vi "Create Top Level.vi"(9 "Alias":string, 10 "Actor":refnum<class "Actor.lvclass">) -> ()   [LabVIEW 2021, in "LVCAM.lvlib" / "Self Actor.lvclass"]
uses:
  Self Actor.lvclass
  Actor/Actor.lvclass
  Self Actor.lvclass/Self Actor.ctl
  LVCAM.lvlib
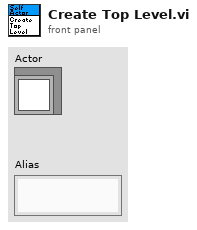
[diagram p1: front panel]
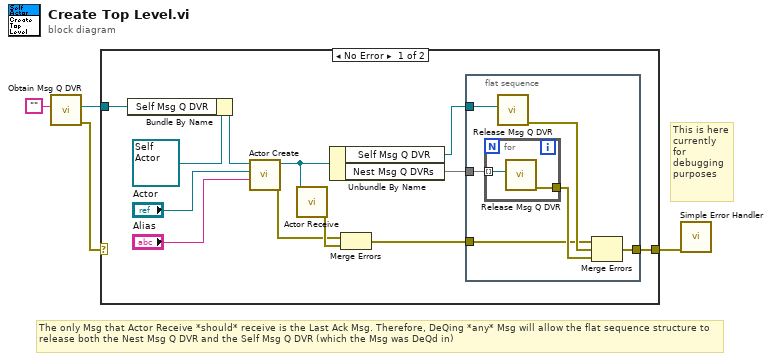
[diagram p0: block diagram]
diagram:
  # "This is here currently for debugging purposes"
  # "The only Msg that Actor Receive *should* receive is the Last Ack Msg. Therefore, DeQing *any* Msg will allow the flat sequence structure to release both the Nest Msg Q DVR and the Self Msg Q DVR (which the Msg was DeQd in)"
  n1 = call "Obtain Msg Q DVR.vi"("Msg Q DVR Alias"="") -> ("error out"=w1:errorcluster, "Msg Q DVR"=w4:refnum<data-value>)  [unwired: 9 in]
  n2 = case shown="No Error" w1 {
    selector: w1 -> [_ w25]
    tunnel: w4 -> [w15 _]
    tunnel: [w14 w25] -> w3
    frame No Error {
      n3 = Bundle By Name(cluster=refnum<class "Self Actor.lvclass"> refnum ("Self Actor in"), "Self Msg Q DVR"=w15) -> (w11:refnum<class "Self Actor.lvclass">)
      n4 = call-dynamic "Actor Create.vi"("Nest Alias"="Alias", "Nest Actor"="Actor", "Self Actor in"=w11) -> ("error out"=w5:errorcluster, "Self Actor out"=w7:refnum<class "Self Actor.lvclass">)  [unwired: 7 in]
      n5 = call-dynamic "Actor Receive.vi"("Self Actor in"=w7) -> ("error out"=w6:errorcluster)  [unwired: 8 in, 2 out]
      n6 = Unbundle By Name(w7) -> ("Self Msg Q DVR"=w16:refnum<data-value>, "Nest Msg Q DVRs"=w13:set{refnum<data-value>})
      n7 = Merge Errors(w5, w6) -> (w12:errorcluster)
      n8 = flat-sequence {
        tunnel: w16 -> [w22]
        tunnel: [w21] -> w14
        tunnel: w13 -> [w20]
        tunnel: w12 -> [w17]
        frame #0 {
          n9 = for {
            tunnel: w20 -> [w24] mode=indexing
            tunnel: [w23] -> w19
            n10 = call "Release Msg Q DVR.vi"("Msg Q DVR"=w24) -> ("error out"=w23:errorcluster)  [unwired: 10 in]
          }
          n11 = call "Release Msg Q DVR.vi"("Msg Q DVR"=w22) -> ("error out"=w18:errorcluster)  [unwired: 10 in]
          n12 = Merge Errors(w17, w18, w19) -> (w21:errorcluster)
        }
      }
    }
    frame Error {
    }
  }
  n13 = call <vilib>:"Simple Error Handler.vi"("error in (no error)"=w3) -> ()  [unwired: 4 in, 5 out]
